vi "Organize PID Outputs.vi"(11 "PID":T1) -> (2 "Gains":cluster{"P":dbl, "I":dbl, "D":dbl}, 3 "Output Range":cluster{"max":dbl, "min":dbl})   [LabVIEW 2013]
uses:
  Common Code/Dashboard UDP/PID Params.ctl
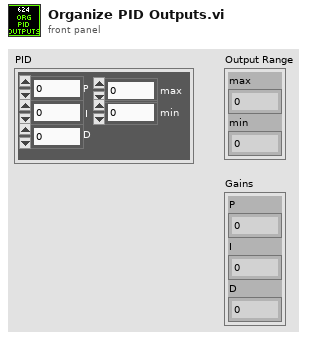
[diagram p1: front panel]
types:
  T1 = typedef "PID Params.ctl" = cluster{"max":dbl, "min":dbl, "P":dbl, "I":dbl, "D":dbl}
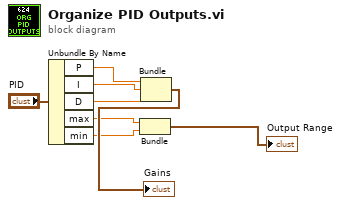
[diagram p0: block diagram]
diagram:
  n1 = Unbundle By Name("PID") -> ("P"=w2:dbl, "I"=w3:dbl, "D"=w4:dbl, "max"=w5:dbl, "min"=w6:dbl)
  n2 = Bundle("max"=w5, "min"=w6) -> (→"Output Range":cluster{"max":dbl, "min":dbl})  [unwired: 1 in]
  n3 = Bundle("P"=w2, "I"=w3, "D"=w4) -> (→"Gains":cluster{"P":dbl, "I":dbl, "D":dbl})  [unwired: 1 in]
